vi "ORS_GalvoConfig3D_v2.vi"(0 "Galvo":T1={"x mirror"="", "y mirror"="", "trig out"="", "x mirror task"="", "y mirror task"="", "trig out task"="", "n_axis"=0, "params"={"n_lines"=512, "n_frames"=1, "force to zero"=FALSE, "Triggers_per_sweep"=0.0, "X center"=0.0, "X span"=0.0, "Y center"=0.0, "Y span"=0.0, "flyb.lines"=0, "n_triggers"=0, "mode"=0, "offset"=5.0, "galvo phase"=0, "span factor"=1.0, "Custom trig."={"n_f to c. trig"=150, "c. trig length"=8, "c. trig interval"=1024, "n_c. trig"=1}, "f_per_pos"=1, "n_dataset"=1, "flyback fr"=1}, "acq trig out"="", "acq trig out task"="", "sample array X"=[], "sample array Y"=[], "custom trig out"="Dev1/port0/line7", "custom trig out task"="", "FDML-box"="TCPIP0::10.153.218.51::23::SOCKET", "ACQ/Galvo"=enum."ADC/FDML", "acq trig out an task"="", "acq trig out an"="", "Galvo Trig input"="", "Galvo Clk input"="", "sample array Acq trig out an"=[]} {"params"."n_dataset" min=1; "params"."X center" format="%^_3g"; "params"."X span" format="%^_3g"; "params"."Y center" format="%^_3g"; "params"."Y span" format="%^_3g"}, 4 "use_digi_trig":bool, 9 "error in":errorcluster) -> (14 "Galvo out":T1={"x mirror"="", "y mirror"="", "trig out"="", "x mirror task"="", "y mirror task"="", "trig out task"="", "n_axis"=0, "params"={"n_lines"=512, "n_frames"=1, "force to zero"=FALSE, "Triggers_per_sweep"=0.0, "X center"=0.0, "X span"=0.0, "Y center"=0.0, "Y span"=0.0, "flyb.lines"=0, "n_triggers"=0, "mode"=0, "offset"=5.0, "galvo phase"=0, "span factor"=1.0, "Custom trig."={"n_f to c. trig"=150, "c. trig length"=8, "c. trig interval"=1024, "n_c. trig"=1}, "f_per_pos"=1, "n_dataset"=1, "flyback fr"=1}, "acq trig out"="", "acq trig out task"="", "sample array X"=[], "sample array Y"=[], "custom trig out"="Dev1/port0/line7", "custom trig out task"="", "FDML-box"="TCPIP0::10.153.218.51::23::SOCKET", "ACQ/Galvo"=enum."ADC/FDML", "acq trig out an task"="", "acq trig out an"="", "Galvo Trig input"="", "Galvo Clk input"="", "sample array Acq trig out an"=[]} {"params"."n_dataset" min=1; "params"."X center" format="%^_3g"; "params"."X span" format="%^_3g"; "params"."Y center" format="%^_3g"; "params"."Y span" format="%^_3g"}, 19 "error out":errorcluster)   [LabVIEW 2021]
uses:
  Typedefs/ORS_Galvo.ctl
  Typedefs/ORS_Galvo_params.ctl
  <vilib>/DAQmx/create/channels.llb/DAQmx Create Channel (DO-Digital Output).vi
  <vilib>/DAQmx/create/channels.llb/DAQmx Create Channel (AO-Voltage-Basic).vi
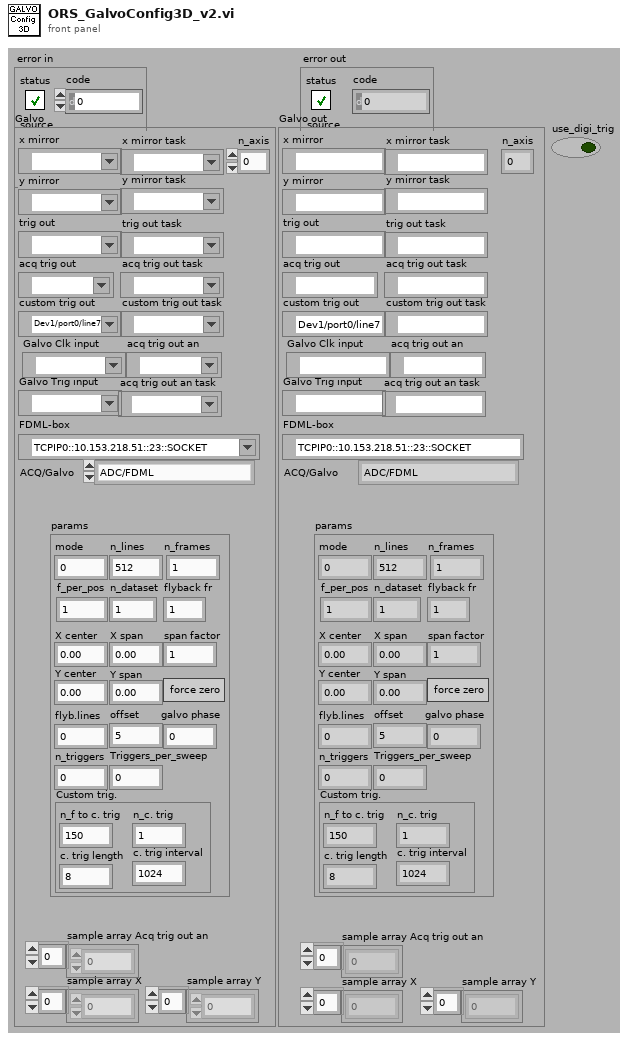
[diagram p1: front panel]
types:
  T1 = typedef "ORS_Galvo.ctl" = cluster{"x mirror":tag, "y mirror":tag, "trig out":tag, "x mirror task":refnum<k21>, "y mirror task":refnum<k21>, "trig out task":refnum<k21>, "n_axis":i32, "params":T2, "acq trig out":tag, "acq trig out task":refnum<k21>, "sample array X":dbl[], "sample array Y":dbl[], "custom trig out":tag, "custom trig out task":refnum<k21>, "FDML-box":refnum<visa-resource-name>, "ACQ/Galvo":enum16{"ADC/FDML", "NI_DAQ", "ADC"}, "acq trig out an task":refnum<k21>, "acq trig out an":tag, "Galvo Trig input":tag, "Galvo Clk input":tag, "sample array Acq trig out an":dbl[]}
  T2 = typedef "ORS_Galvo_params.ctl" = cluster{"n_lines":i32, "n_frames":i32, "force to zero":bool, "Triggers_per_sweep":dbl, "X center":dbl, "X span":dbl, "Y center":dbl, "Y span":dbl, "flyb.lines":i32, "n_triggers":i32, "mode":i32, "offset":dbl, "galvo phase":i32, "span factor":dbl, "Custom trig.":cluster{"n_f to c. trig":i32, "c. trig length":i32, "c. trig interval":i32, "n_c. trig":i32}, "f_per_pos":i32, "n_dataset":u32, "flyback fr":u16}
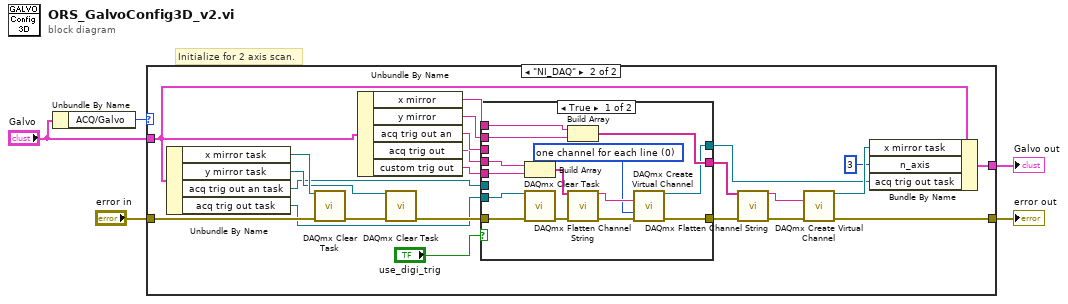
[diagram p0: block diagram]
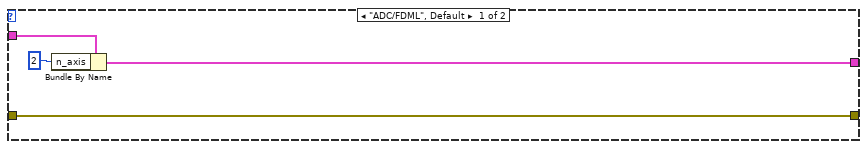
[diagram p2: hidden frame]
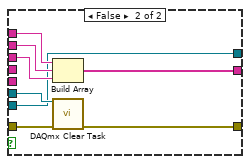
[diagram p3: hidden frame]
diagram:
  # "Initialize for 2 axis scan."
  n1 = Unbundle By Name("Galvo") -> ("ACQ/Galvo"=w1:enum16{"ADC/FDML", "NI_DAQ", "ADC"})
  n2 = case shown="\"NI_DAQ\"" w1 {
    tunnel: "error in" -> [w9 w32]
    tunnel: [w9 w22] -> w4
    tunnel: [w7 w20] -> w3
    tunnel: "Galvo" -> [w8 w19]
    frame "ADC/FDML", Default {
      n3 = Bundle By Name(cluster=w8, "n_axis"=2) -> (w7:T1)
    }
    frame "NI_DAQ" {
      n4 = Unbundle By Name(w19) -> ("x mirror task"=w26:refnum<k21>, "y mirror task"=w25:refnum<k21>, "acq trig out an task"=w17:refnum<k21>, "acq trig out task"=w13:refnum<k21>)
      n5 = call <vilib>:"DAQmx Clear Task.vi"("task in"=w26, "error in"=w32) -> ("error out"=w24:errorcluster)  [unwired: 13 in]
      n6 = Unbundle By Name(w19) -> ("x mirror"=w30:tag, "y mirror"=w31:tag, "acq trig out an"=w18:tag, "acq trig out"=w11:tag, "custom trig out"=w10:tag)
      n7 = call <vilib>:"DAQmx Clear Task.vi"("task in"=w25, "error in"=w24) -> ("error out"=w16:errorcluster)  [unwired: 13 in]
      n8 = case shown="True" "use_digi_trig" {
        tunnel: w31 -> [w46 w54]
        tunnel: w30 -> [w45 w53]
        tunnel: [w44 w52] -> w29
        tunnel: w18 -> [_ w51]
        tunnel: w17 -> [_ w50]
        tunnel: w16 -> [w43 w49]
        tunnel: [w39 w48] -> w15
        tunnel: w13 -> [w42 w47]
        tunnel: [w38 w47] -> w12
        tunnel: w11 -> [w37 _]
        tunnel: w10 -> [w36 _]
        frame True {
          w33 = 0 items=["one channel for each line", "one channel for all lines"] ("line grouping")
          n9 = Build Array(w37, w36) -> (w35:tag[])
          n10 = call <vilib>:"DAQmx Clear Task.vi"("task in"=w42, "error in"=w43) -> ("error out"=w41:errorcluster)  [unwired: 13 in]
          n11 = Build Array(w45, w46) -> (w44:tag[])
          n12 = call <vilib>:"DAQmx Flatten Channel String.vi"("names in"=w35, "error in"=w41) -> ("names out"=w34:string, "error out"=w40:errorcluster)  [unwired: 12 in]
          n13 = call-poly <vilib>:"DAQmx Create Virtual Channel.vi"("lines"=w34, "line grouping"=w33, "error in"=w40) -> ("task out"=w38:refnum<k21>, "error out"=w39:errorcluster)  [unwired: 11 in]
        }
        frame False {
          n14 = Build Array(w53, w54, w51) -> (w52:tag[])
          n15 = call <vilib>:"DAQmx Clear Task.vi"("task in"=w50, "error in"=w49) -> ("error out"=w48:errorcluster)  [unwired: 13 in]
        }
      }
      n16 = call <vilib>:"DAQmx Flatten Channel String.vi"("names in"=w29, "error in"=w15) -> ("names out"=w28:string, "error out"=w27:errorcluster)  [unwired: 12 in]
      n17 = call-poly <vilib>:"DAQmx Create Virtual Channel.vi"("physical channels"=w28, "error in"=w27) -> ("task out"=w23:refnum<k21>, "error out"=w22:errorcluster)  [unwired: 12 in]
      n18 = Bundle By Name(cluster=w19, "x mirror task"=w23, "n_axis"=3, "acq trig out task"=w12) -> (w20:T1)
    }
  }
  "error out" <- w4
  "Galvo out" <- w3
